vi "Event Handler.vi"(0 "Event Id":string, 5 "Data":variant, 11 "error in (no error)":errorcluster, 13 "Operation":T1) -> (4 "Event Reference":refnum<user-event>, 15 "error out":errorcluster)   [LabVIEW 2019, in "STS_LTRV.lvlib"]
uses:
  STS_LTRV.lvlib
  TypeDefs/Event Handler/Operation.ctl
  TypeDefs/Event Handler/Event Data.ctl
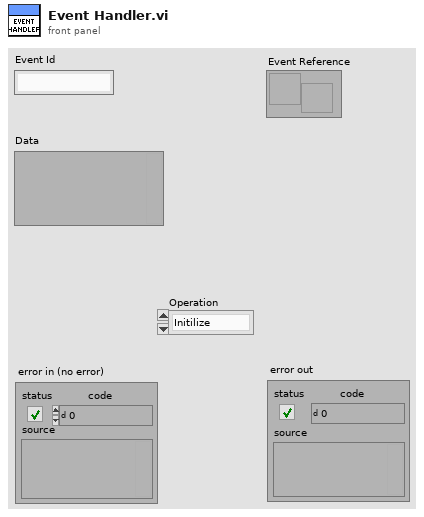
[diagram p1: front panel]
types:
  T1 = typedef "STS_LTRV.lvlib/Operation.ctl" = enum16{"Initilize", "Get Reference", "Publish", "Destroy"}
  T2 = typedef "STS_LTRV.lvlib/Event Data.ctl" = cluster{"Event":string, "Data":variant}
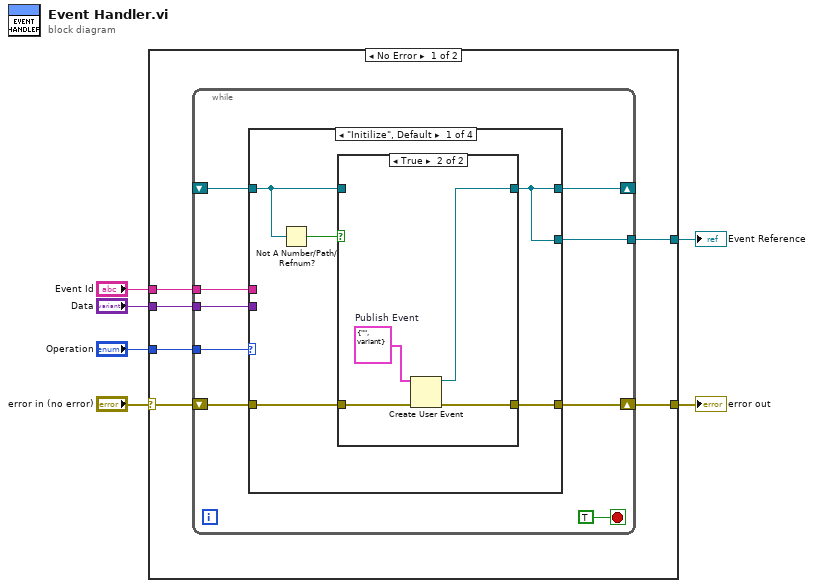
[diagram p0: block diagram]
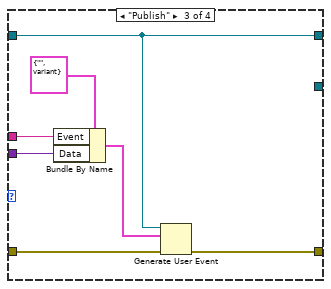
[diagram p4: hidden frame]
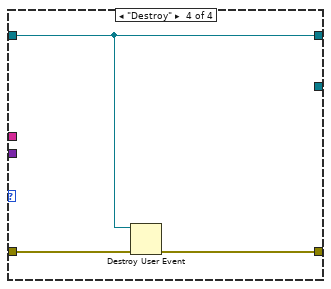
[diagram p5: hidden frame]
diagram:
  n1 = case shown="No Error" "error in (no error)" {
    selector: "error in (no error)" -> [w12 w45]
    tunnel: "Operation" -> [w11 _]
    tunnel: [w10 w45] -> w4
    tunnel: "Event Id" -> [w9 _]
    tunnel: "Data" -> [w8 _]
    tunnel: [w7 _] -> w1
    frame No Error {
      n2 = while {
        shift-right: [w19] -> w10
        shift-left: w12 -> [w21]
        tunnel: w11 -> [w20]
        tunnel: w9 -> [w18]
        tunnel: w8 -> [w17]
        shift-right: [w15] -> _
        shift-left: _ -> [w14]
        tunnel: [w13] -> w7
        stop <- TRUE stop-if-true
        n3 = case shown="\"Initilize\", Default" w20 {
          tunnel: w21 -> [w26 w34 w40 w43]
          tunnel: [w25 w34 w41 w44] -> w19
          tunnel: w18 -> [_ _ w38 _]
          tunnel: w17 -> [_ _ w37 _]
          tunnel: [w22 w33 w35 w42] -> w15
          tunnel: w14 -> [w23 w33 w35 w42]
          tunnel: [w22 w33 _ _] -> w13
          frame "Initilize", Default {
            n4 = Not A Number/Path/Refnum?(number/path/refnum=w23) -> (NaN/Path/Refnum?=w24:bool)
            n5 = case shown="True" w24 {
              tunnel: w26 -> [w28 w32]
              tunnel: [w28 w30] -> w25
              tunnel: [w27 w29] -> w22
              tunnel: w23 -> [w27 _]
              frame False {
              }
              frame True {
                w31 = T2 {"Event"="", "Data"=variant}  # Publish Event
                n6 = Create User Event(user event datatype=w31, error in=w32) -> (user event=w29:refnum<user-event>, error out=w30:errorcluster)
              }
            }
          }
          frame "Get Reference" {
          }
          frame "Publish" {
            n7 = Bundle By Name(cluster=T2 {"Event"="", "Data"=variant}, "Event"=w38, "Data"=w37) -> (w36:T2)
            n8 = Generate User Event(user event=w35, event data cluster=w36, error in=w40) -> (error out=w41:errorcluster)  [unwired: 1 in, 1 out]
          }
          frame "Destroy" {
            n9 = Destroy User Event(user event=w42, error in=w43) -> (error out=w44:errorcluster)
          }
        }
      }
    }
    frame Error {
    }
  }
  "error out" <- w4
  "Event Reference" <- w1
